vi "re_LuaVIEW Call.vi"(0 "function name":string, 5 "LuaVIEW reference in":T1, 7 "required results (no checking needed)":i32=-1, 11 "error in (no error)":errorcluster) -> (6 "LuaVIEW reference out":T1, 15 "error out":errorcluster)   [LabVIEW 2013]
doc: "Call a Lua-side function. Any elements pushed onto the stack prior to the call are passed as arguments. When the function returns, the stack holds the function result values, if any. The call is protected so that any errors during the function's execution are caught.\nNever make simultaneous calls to the same LuaVIEW state.\n\nTo be able to make Lua-side calls, open a LuaVIEW base state using \"Open Base State\" and compile one or more scripts implementing the function or functions to be called using \"Compile\". Next, the resulting compilations must be executed using \"Execute\" so that the functions become defined. After that, \"Call\" can be used on all defined functions. Functions called via \"Call\" cannot call LabVIEW-side functions and are not interruptable other than through throwing an error."
uses:
  typedefs/t_LuaVIEW Reference.ctl
  typedefs/et_LuaVIEW CIN Actions.ctl
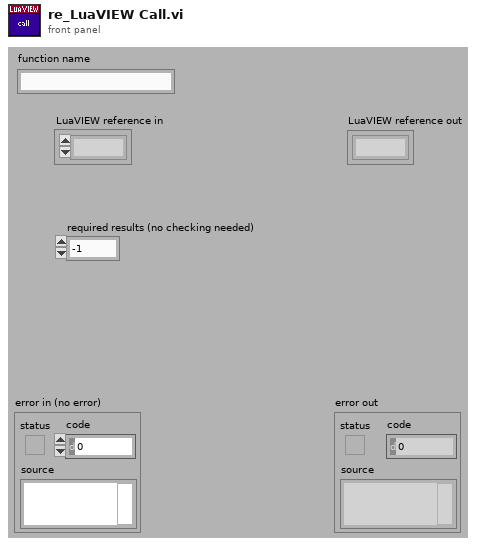
[diagram p1: front panel]
types:
  T1 = typedef "t_LuaVIEW Reference.ctl" = refnum<k1>
  T2 = typedef "et_LuaVIEW CIN Actions.ctl" = enum16{"checksynopsis", "_open", "_registerpublic", "_registerexport", "__never_an_error_result_ns", "luaversion", "cinversion", "_totals", "_taskcount", "pathological", "_unregnextpublic", "registryusecount", "__per_state_actions", "regsetprivate", "regsetindex", "regsetmodule", "_revokeexports", "_usepublic", "prepare", "compile", "execute", "call", "unregstaterefs", "_close", "pullboolean", "pullnumber", "pullI8", "pullU8", "pullI16", "pullU16", "pullI32", "pullU32", "pullobject", "pullrefnum", "pullstring", "pullflat", "pushflat", "pushobject", "getattribute", "setattribute", "stacktostring", "_startyieldtest", "_endyieldtest", "_pollprintbuffer", "__never_an_error_result_ps", "_pollexport", "setclone", "forcecleanup", "gettop", "clearstack", "insert", "pushboolean", "pushnumber", "pushrefnum", "pushstring", "pushnil", "pushvalue", "gettaskref", "settaskref"}
  T3 = typedef "et_LuaVIEW CIN Results.ctl" = enum16{"OK", "error", "main", "call", "clonecall", "modulecall", "exportcall", "index", "yield"}
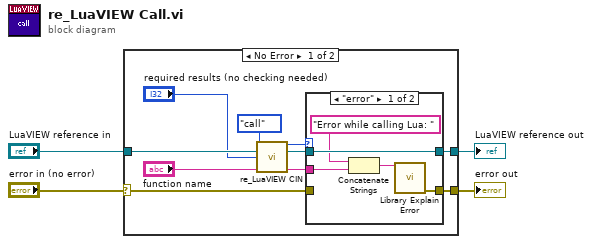
[diagram p0: block diagram]
diagram:
  n1 = case shown="No Error" "error in (no error)" {
    selector: "error in (no error)" -> [w8 w23]
    tunnel: [w7 w22] -> w4
    tunnel: [w14 w23] -> w3
    tunnel: "LuaVIEW reference in" -> [w13 w22]
    frame No Error {
      n2 = call "re_LuaVIEW CIN.vi"("action"=et_LuaVIEW_CIN_Actions."call", "LuaVIEW reference in"=w13, "index in"="required results (no checking needed)", "string in"="function name") -> ("result"=w11:T3, "LuaVIEW reference out"=w9:T1, "string out"=w10:string)  [unwired: 5 in, 4 out]
      n3 = case shown="\"error\"" w11 {
        tunnel: w10 -> [w16 _]
        tunnel: [w19 w20] -> w14
        tunnel: w9 -> [w18 w21]
        tunnel: [w18 w21] -> w7
        tunnel: w8 -> [_ w20]
        frame "error" {
          n4 = Concatenate Strings("Error while calling Lua: " ("string"), w16) -> (w17:string)
          n5 = call "Library Explain Error.vi"("explanation prefix (none)"=w17) -> ("explained error"=w19:errorcluster)  [unwired: 14 in]
        }
        frame Default {
        }
      }
    }
    frame Error {
    }
  }
  "LuaVIEW reference out" <- w4
  "error out" <- w3
